vi "Lift State Machine.vi"() -> ()   [LabVIEW 2014]
uses:
  Global Variables.vi
panel:
  in  "Lift Speed 2":dbl=0.25 format="%#_13g"
  in  "Distance Down":dbl=6.0 format="%#_13g"
  in  "Distance Back Up":dbl=6.0 format="%#_13g"
  in  "Lift Speed":dbl=3.0
  in  "Offset":u32=3
  in  "Offset Step":bool
  out "State":i32=3
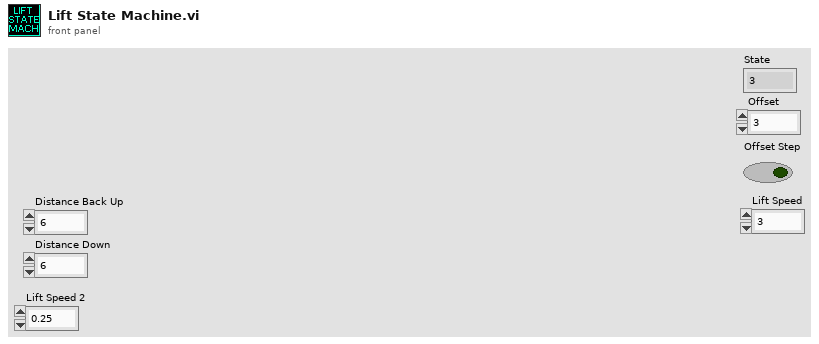
[diagram p1: front panel]
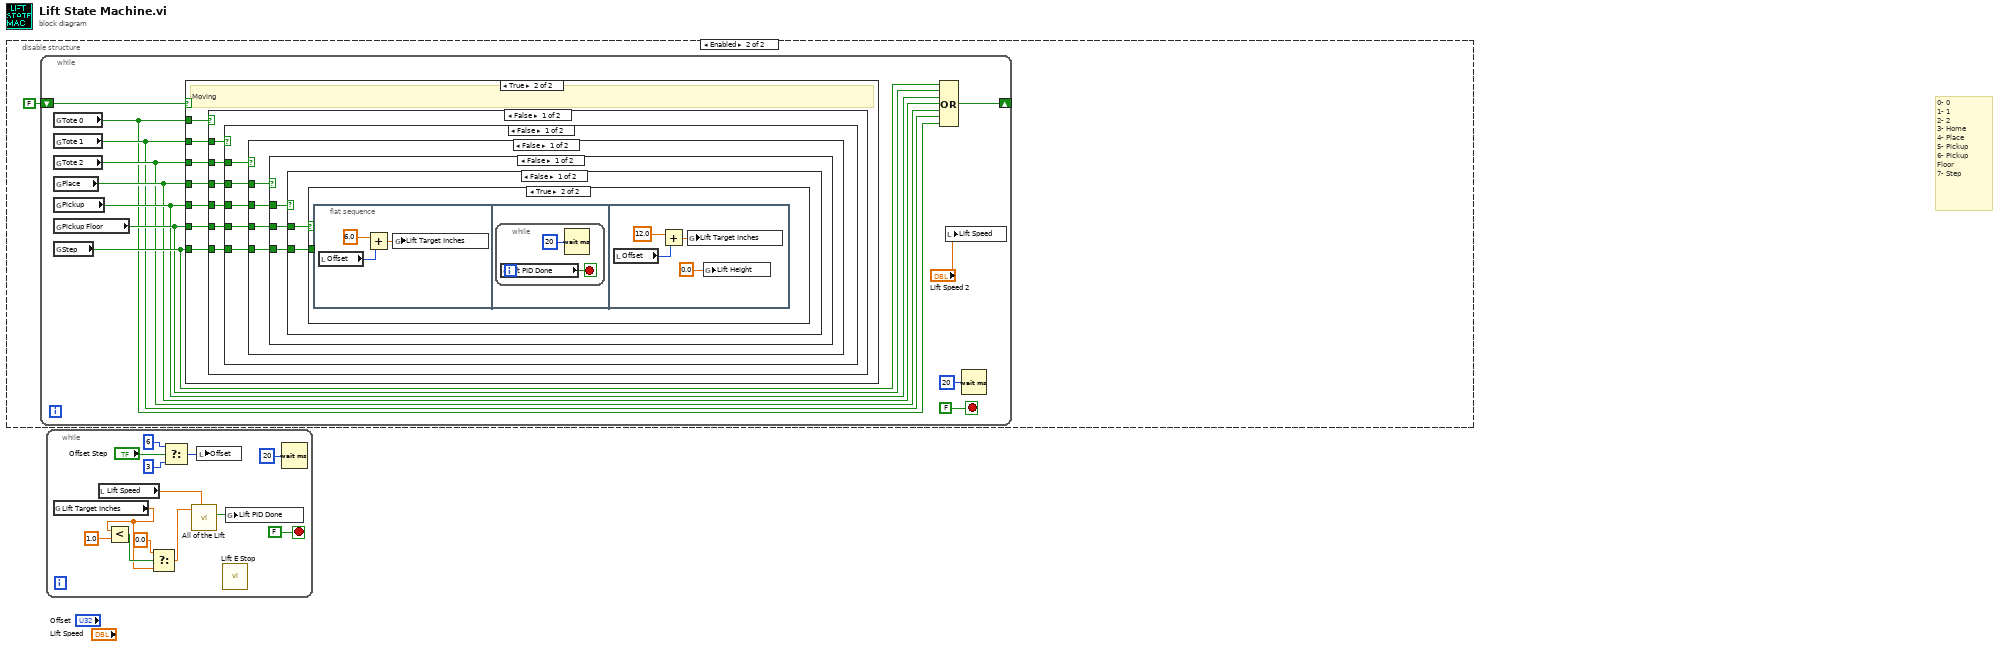
[diagram p0: block diagram]
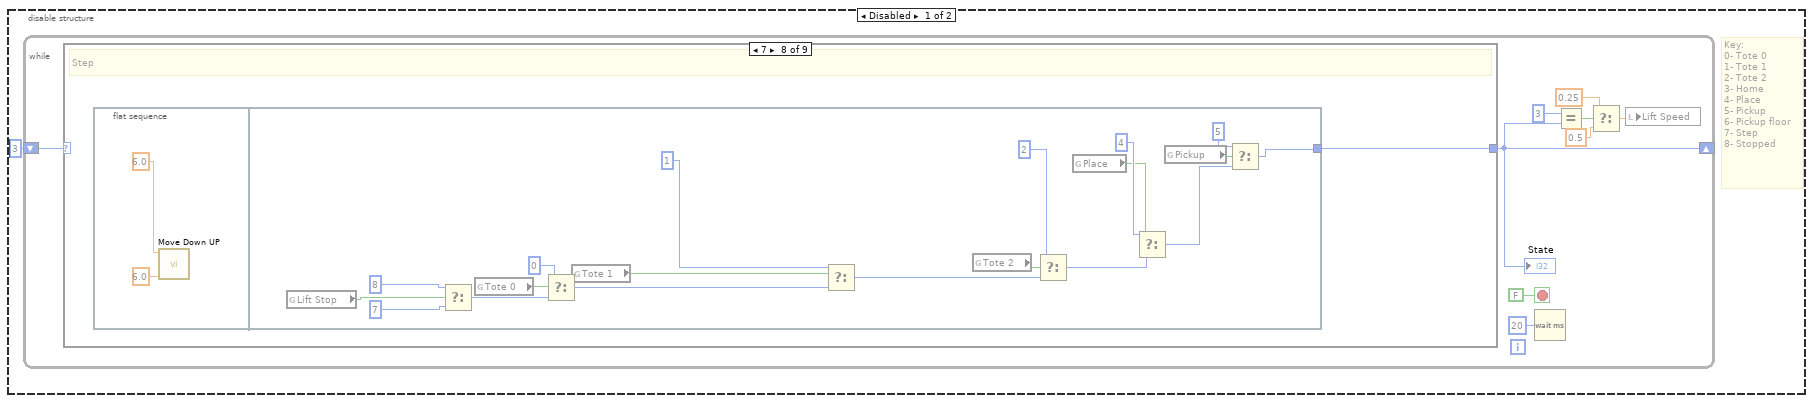
[diagram p2: hidden frame]
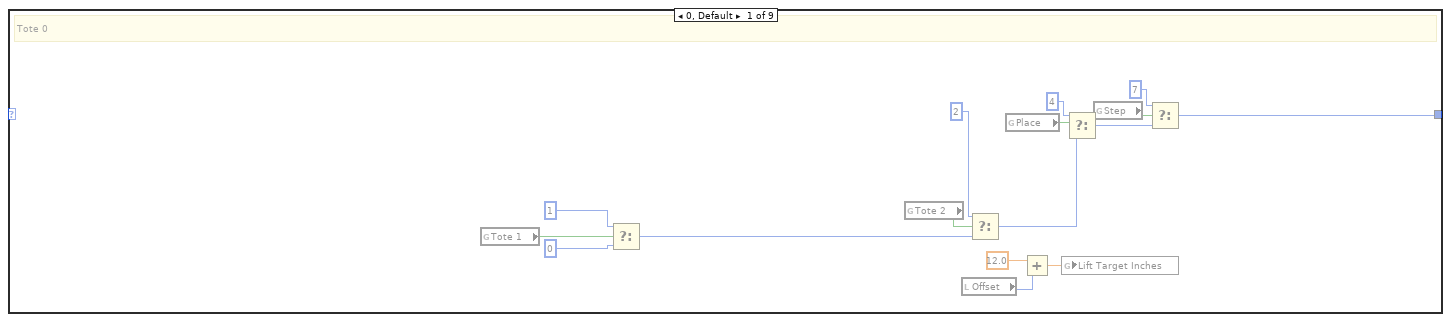
[diagram p3: hidden frame]
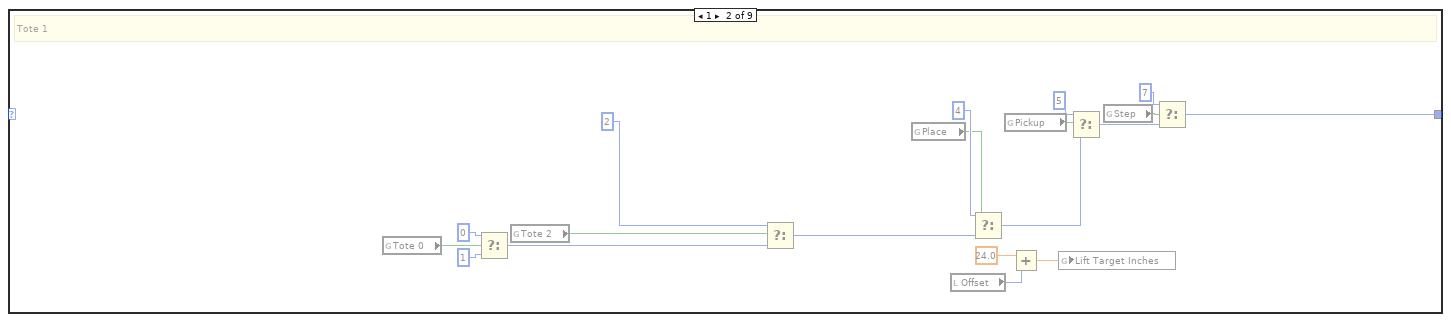
[diagram p4: hidden frame]
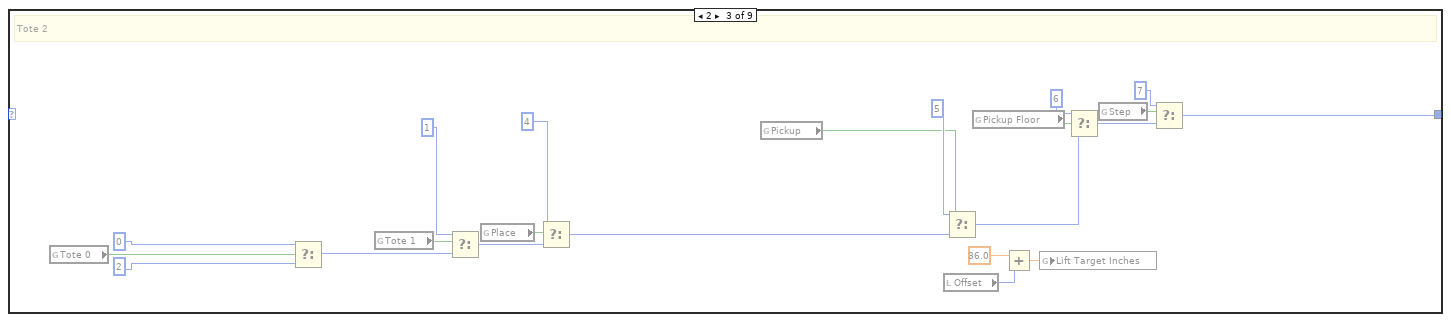
[diagram p5: hidden frame]
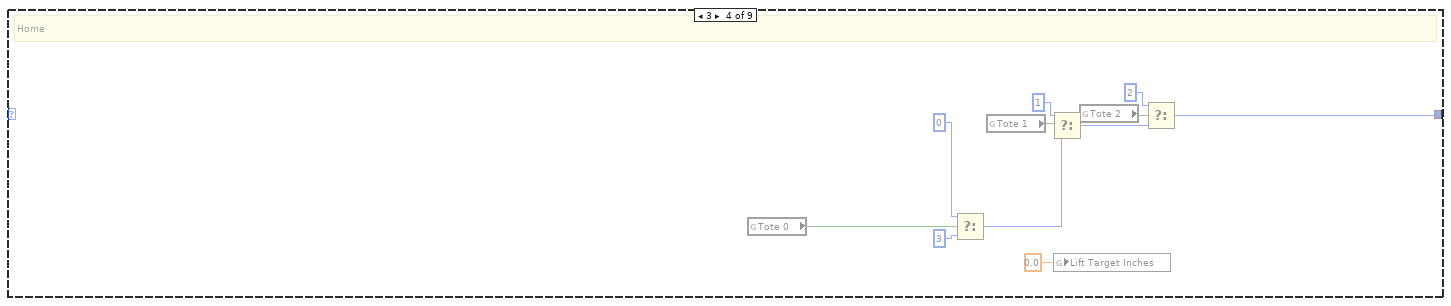
[diagram p6: hidden frame]
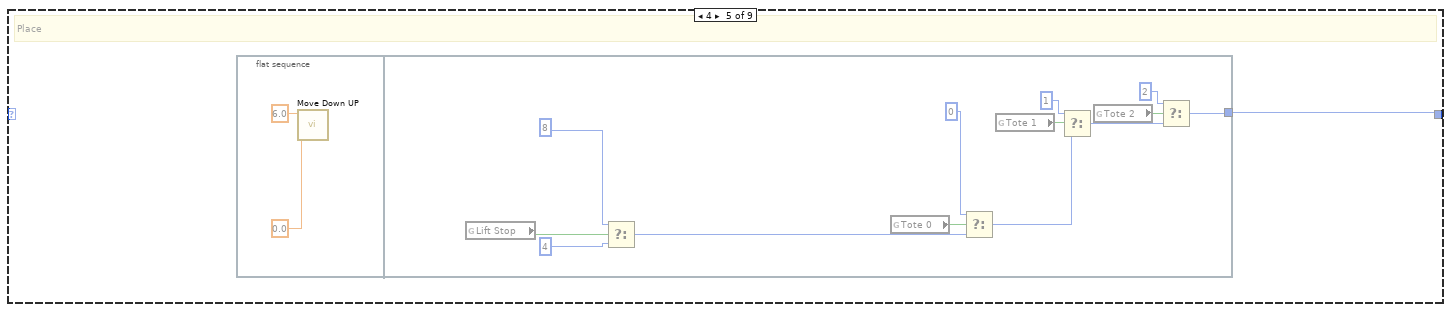
[diagram p7: hidden frame]
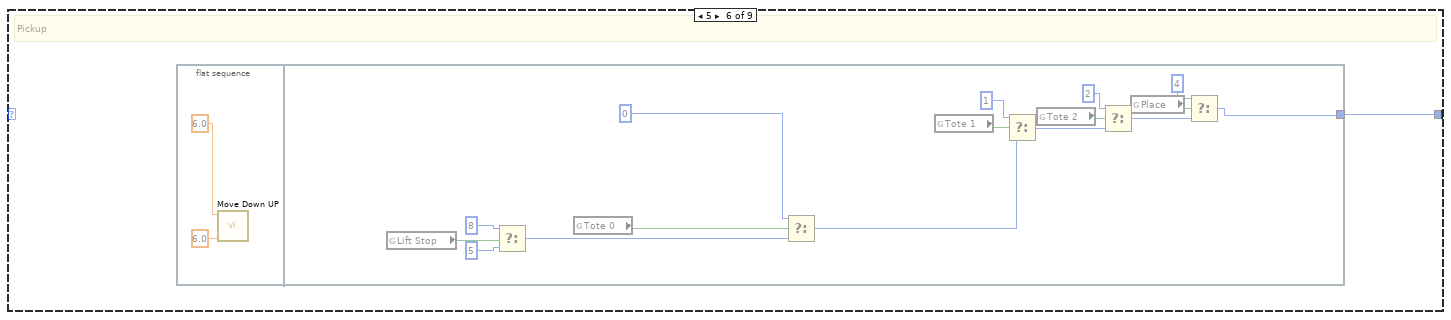
[diagram p8: hidden frame]
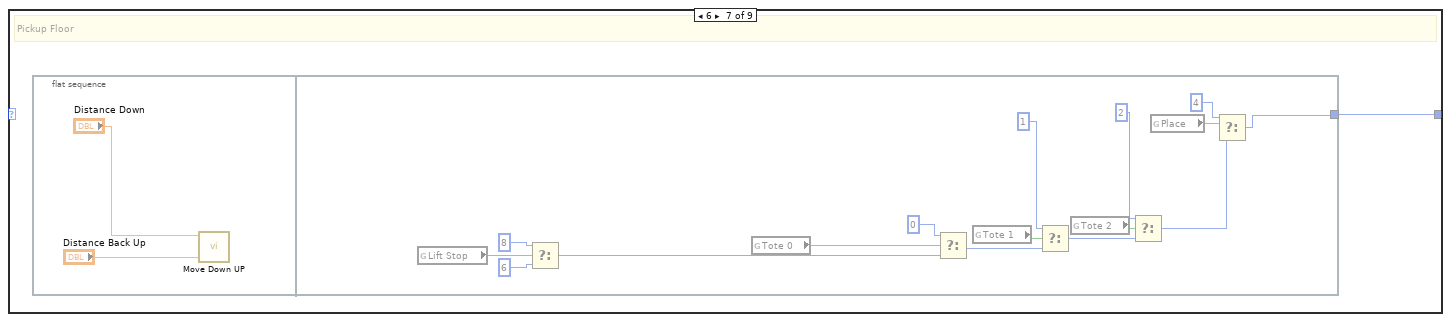
[diagram p9: hidden frame]
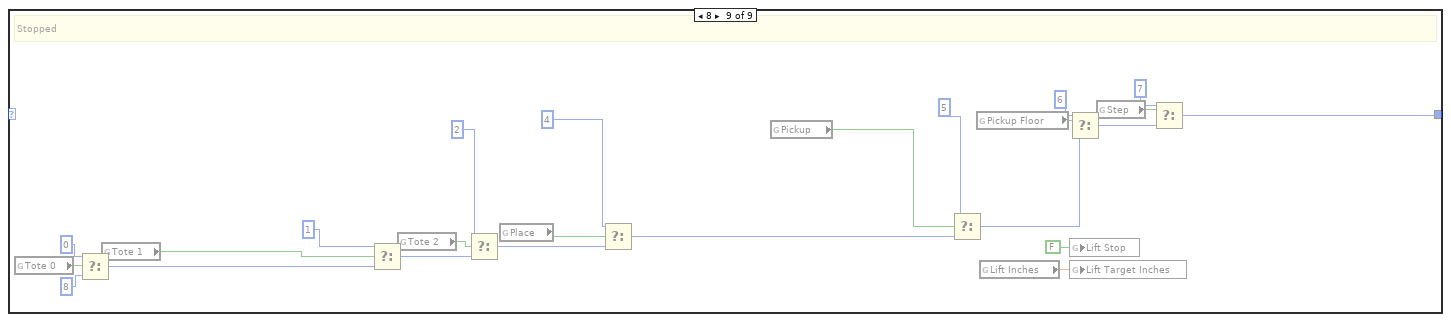
[diagram p10: hidden frame]
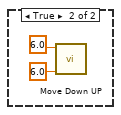
[diagram p13: hidden frame]
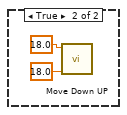
[diagram p14: hidden frame]
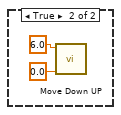
[diagram p15: hidden frame]
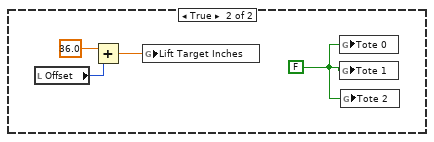
[diagram p16: hidden frame]
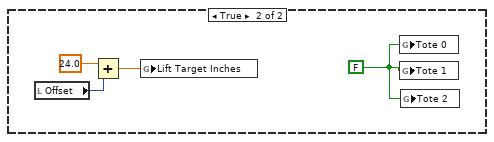
[diagram p17: hidden frame]
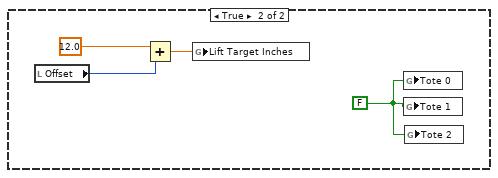
[diagram p18: hidden frame]
diagram:
  # "0- 0\n1- 1\n2- 2\n3- Home\n4- Place\n5- Pickup\n6- Pickup Floor\n7- Step"
  n1 = disable-structure shown="Enabled" {
    frame Disabled {
      # "Key:\n0- Tote 0\n1- Tote 1\n2- Tote 2\n3- Home\n4- Place\n5- Pickup\n6- Pickup floor\n7- Step\n8- Stopped"
      n2 = while {
        shift-right: [w6] -> _
        shift-left: 3 ("f") -> [w10]
        stop <- FALSE stop-if-true
        n3 = case shown="7" w10 {
          tunnel: [w19 w40 w63 w72 w79 w95 w114 w133 w156] -> w6
          frame 0, Default {
            # "Tote 0"
            n4 = global read "Global Variables.vi" "Tote 1"() -> (w15:bool)
            n5 = Select(t=1, s=w15, f=0) -> (s? t:f=w23:i32)
            n6 = global read "Global Variables.vi" "Tote 2"() -> (w14:bool)
            n7 = local read "Offset"() -> (w16:u32)
            n8 = Select(t=2, s=w14, f=w23) -> (s? t:f=w20:i32)
            n9 = global read "Global Variables.vi" "Place"() -> (w13:bool)
            n10 = Add(x=12.0, y=w16) -> (x+y=w11:dbl)
            n11 = global write "Global Variables.vi" "Lift Target Inches"(w11) -> ()
            n12 = Select(t=4, s=w13, f=w20) -> (s? t:f=w18:i32)
            n13 = global read "Global Variables.vi" "Step"() -> (w12:bool)
            n14 = Select(t=7, s=w12, f=w18) -> (s? t:f=w19:i32)
          }
          frame 1 {
            # "Tote 1"
            n15 = global read "Global Variables.vi" "Tote 0"() -> (w32:bool)
            n16 = Select(t=0, s=w32, f=1) -> (s? t:f=w37:i32)
            n17 = global read "Global Variables.vi" "Tote 2"() -> (w31:bool)
            n18 = Select(t=2, s=w31, f=w37) -> (s? t:f=w36:i32)
            n19 = global read "Global Variables.vi" "Place"() -> (w30:bool)
            n20 = local read "Offset"() -> (w33:u32)
            n21 = Select(t=4, s=w30, f=w36) -> (s? t:f=w39:i32)
            n22 = global read "Global Variables.vi" "Pickup"() -> (w29:bool)
            n23 = Add(x=24.0, y=w33) -> (x+y=w27:dbl)
            n24 = global write "Global Variables.vi" "Lift Target Inches"(w27) -> ()
            n25 = Select(t=5, s=w29, f=w39) -> (s? t:f=w35:i32)
            n26 = global read "Global Variables.vi" "Step"() -> (w28:bool)
            n27 = Select(t=7, s=w28, f=w35) -> (s? t:f=w40:i32)
          }
          frame 2 {
            # "Tote 2"
            n28 = global read "Global Variables.vi" "Tote 0"() -> (w53:bool)
            n29 = Select(t=0, s=w53, f=2) -> (s? t:f=w61:i32)
            n30 = global read "Global Variables.vi" "Tote 1"() -> (w52:bool)
            n31 = Select(t=1, s=w52, f=w61) -> (s? t:f=w59:i32)
            n32 = global read "Global Variables.vi" "Place"() -> (w48:bool)
            n33 = Select(t=4, s=w48, f=w59) -> (s? t:f=w57:i32)
            n34 = global read "Global Variables.vi" "Pickup"() -> (w47:bool)
            n35 = local read "Offset"() -> (w54:u32)
            n36 = Select(t=5, s=w47, f=w57) -> (s? t:f=w56:i32)
            n37 = global read "Global Variables.vi" "Pickup Floor"() -> (w51:bool)
            n38 = Add(x=36.0, y=w54) -> (x+y=w49:dbl)
            n39 = global write "Global Variables.vi" "Lift Target Inches"(w49) -> ()
            n40 = Select(t=6, s=w51, f=w56) -> (s? t:f=w66:i32)
            n41 = global read "Global Variables.vi" "Step"() -> (w50:bool)
            n42 = Select(t=7, s=w50, f=w66) -> (s? t:f=w63:i32)
          }
          frame 3 {
            # "Home"
            n43 = global read "Global Variables.vi" "Tote 0"() -> (w71:bool)
            n44 = Select(t=0, s=w71, f=3) -> (s? t:f=w74:i32)
            n45 = global read "Global Variables.vi" "Tote 1"() -> (w70:bool)
            n46 = Select(t=1, s=w70, f=w74) -> (s? t:f=w77:i32)
            n47 = global write "Global Variables.vi" "Lift Target Inches"(0.0 ("x")) -> ()
            n48 = global read "Global Variables.vi" "Tote 2"() -> (w69:bool)
            n49 = Select(t=2, s=w69, f=w77) -> (s? t:f=w72:i32)
          }
          frame 4 {
            # "Place"
            n50 = flat-sequence {
              tunnel: [w82] -> w79
              frame #0 {
                n51 = call "Move Down UP.vi"("Distance Up"=0.0, "Distance Down"=6.0) -> ()  [unwired: 10 in]
              }
              frame #1 {
                n52 = global read "Global Variables.vi" "Lift Stop"() -> (w86:bool)
                n53 = Select(t=8, s=w86, f=4) -> (s? t:f=w83:i32)
                n54 = global read "Global Variables.vi" "Tote 0"() -> (w89:bool)
                n55 = Select(t=0, s=w89, f=w83) -> (s? t:f=w91:i32)
                n56 = global read "Global Variables.vi" "Tote 1"() -> (w88:bool)
                n57 = Select(t=1, s=w88, f=w91) -> (s? t:f=w93:i32)
                n58 = global read "Global Variables.vi" "Tote 2"() -> (w87:bool)
                n59 = Select(t=2, s=w87, f=w93) -> (s? t:f=w82:i32)
              }
            }
          }
          frame 5 {
            # "Pickup"
            n60 = flat-sequence {
              tunnel: [w98] -> w95
              frame #0 {
                n61 = call "Move Down UP.vi"("Distance Up"=6.0, "Distance Down"=6.0) -> ()  [unwired: 10 in]
              }
              frame #1 {
                n62 = global read "Global Variables.vi" "Lift Stop"() -> (w102:bool)
                n63 = Select(t=8, s=w102, f=5) -> (s? t:f=w99:i32)
                n64 = global read "Global Variables.vi" "Tote 0"() -> (w106:bool)
                n65 = Select(t=0, s=w106, f=w99) -> (s? t:f=w107:i32)
                n66 = global read "Global Variables.vi" "Tote 1"() -> (w105:bool)
                n67 = Select(t=1, s=w105, f=w107) -> (s? t:f=w110:i32)
                n68 = global read "Global Variables.vi" "Tote 2"() -> (w104:bool)
                n69 = Select(t=2, s=w104, f=w110) -> (s? t:f=w109:i32)
                n70 = global read "Global Variables.vi" "Place"() -> (w103:bool)
                n71 = Select(t=4, s=w103, f=w109) -> (s? t:f=w98:i32)
              }
            }
          }
          frame 6 {
            # "Pickup Floor"
            n72 = flat-sequence {
              tunnel: [w118] -> w114
              frame #0 {
                n73 = call "Move Down UP.vi"("Distance Up"="Distance Back Up", "Distance Down"="Distance Down") -> ()  [unwired: 10 in]
              }
              frame #1 {
                n74 = global read "Global Variables.vi" "Lift Stop"() -> (w119:bool)
                n75 = Select(t=8, s=w119, f=6) -> (s? t:f=w120:i32)
                n76 = global read "Global Variables.vi" "Tote 0"() -> (w126:bool)
                n77 = Select(t=0, s=w126, f=w120) -> (s? t:f=w127:i32)
                n78 = global read "Global Variables.vi" "Tote 1"() -> (w125:bool)
                n79 = Select(t=1, s=w125, f=w127) -> (s? t:f=w130:i32)
                n80 = global read "Global Variables.vi" "Tote 2"() -> (w124:bool)
                n81 = Select(t=2, s=w124, f=w130) -> (s? t:f=w129:i32)
                n82 = global read "Global Variables.vi" "Place"() -> (w123:bool)
                n83 = Select(t=4, s=w123, f=w129) -> (s? t:f=w118:i32)
              }
            }
          }
          frame 7 {
            # "Step"
            n84 = flat-sequence {
              tunnel: [w136] -> w133
              frame #0 {
                n85 = call "Move Down UP.vi"("Distance Up"=6.0, "Distance Down"=6.0) -> ()  [unwired: 10 in]
              }
              frame #1 {
                n86 = global read "Global Variables.vi" "Lift Stop"() -> (w137:bool)
                n87 = Select(t=8, s=w137, f=7) -> (s? t:f=w139:i32)
                n88 = global read "Global Variables.vi" "Tote 0"() -> (w145:bool)
                n89 = Select(t=0, s=w145, f=w139) -> (s? t:f=w146:i32)
                n90 = global read "Global Variables.vi" "Tote 1"() -> (w144:bool)
                n91 = Select(t=1, s=w144, f=w146) -> (s? t:f=w150:i32)
                n92 = global read "Global Variables.vi" "Tote 2"() -> (w143:bool)
                n93 = Select(t=2, s=w143, f=w150) -> (s? t:f=w151:i32)
                n94 = global read "Global Variables.vi" "Place"() -> (w142:bool)
                n95 = Select(t=4, s=w142, f=w151) -> (s? t:f=w148:i32)
                n96 = global read "Global Variables.vi" "Pickup"() -> (w141:bool)
                n97 = Select(t=5, s=w141, f=w148) -> (s? t:f=w136:i32)
              }
            }
          }
          frame 8 {
            # "Stopped"
            n98 = global read "Global Variables.vi" "Tote 0"() -> (w158:bool)
            n99 = Select(t=0, s=w158, f=8) -> (s? t:f=w160:i32)
            n100 = global read "Global Variables.vi" "Tote 1"() -> (w163:bool)
            n101 = Select(t=1, s=w163, f=w160) -> (s? t:f=w161:i32)
            n102 = global read "Global Variables.vi" "Tote 2"() -> (w168:bool)
            n103 = Select(t=2, s=w168, f=w161) -> (s? t:f=w169:i32)
            n104 = global read "Global Variables.vi" "Place"() -> (w167:bool)
            n105 = Select(t=4, s=w167, f=w169) -> (s? t:f=w173:i32)
            n106 = global read "Global Variables.vi" "Pickup"() -> (w166:bool)
            n107 = Select(t=5, s=w166, f=w173) -> (s? t:f=w174:i32)
            n108 = global read "Global Variables.vi" "Pickup Floor"() -> (w165:bool)
            n109 = global read "Global Variables.vi" "Lift Inches"() -> (w178:dbl)
            n110 = Select(t=6, s=w165, f=w174) -> (s? t:f=w171:i32)
            n111 = global write "Global Variables.vi" "Lift Stop"(FALSE ("Lift Stop")) -> ()
            n112 = global write "Global Variables.vi" "Lift Target Inches"(w178) -> ()
            n113 = global read "Global Variables.vi" "Step"() -> (w164:bool)
            n114 = Select(t=7, s=w164, f=w171) -> (s? t:f=w156:i32)
          }
        }
        "State" <- w6
        n115 = Wait (ms)(milliseconds to wait=u32 20) -> ()  [unwired: 1 out]
        n116 = Equal?(x=3, y=w6) -> (x = y?=w5:bool)
        n117 = Select(t=0.25, s=w5, f=0.5) -> (s? t:f=w7:dbl)
        n118 = local write "Lift Speed"(w7) -> ()
      }
    }
    frame Enabled {
      n119 = while {
        shift-right: [w182] -> _
        shift-left: FALSE -> [w190]
        stop <- FALSE stop-if-true
        n120 = global read "Global Variables.vi" "Tote 0"() -> (w183:bool)
        n121 = global read "Global Variables.vi" "Tote 1"() -> (w184:bool)
        n122 = global read "Global Variables.vi" "Tote 2"() -> (w185:bool)
        n123 = global read "Global Variables.vi" "Place"() -> (w186:bool)
        n124 = global read "Global Variables.vi" "Pickup"() -> (w187:bool)
        n125 = global read "Global Variables.vi" "Pickup Floor"() -> (w188:bool)
        n126 = global read "Global Variables.vi" "Step"() -> (w189:bool)
        n127 = case shown="True" w190 {
          tunnel: w183 -> [_ w198]
          tunnel: w184 -> [_ w197]
          tunnel: w185 -> [_ w196]
          tunnel: w186 -> [_ w195]
          tunnel: w187 -> [_ w194]
          tunnel: w188 -> [_ w193]
          tunnel: w189 -> [_ w192]
          frame False {
            # "Idling"
          }
          frame True {
            # "Moving"
            n128 = case shown="False" w198 {
              tunnel: w197 -> [w204 _]
              tunnel: w196 -> [w203 _]
              tunnel: w195 -> [w202 _]
              tunnel: w194 -> [w201 _]
              tunnel: w193 -> [w200 _]
              tunnel: w192 -> [w199 _]
              frame False {
                n129 = case shown="False" w204 {
                  tunnel: w203 -> [w209 _]
                  tunnel: w202 -> [w208 _]
                  tunnel: w201 -> [w207 _]
                  tunnel: w200 -> [w206 _]
                  tunnel: w199 -> [w205 _]
                  frame False {
                    n130 = case shown="False" w209 {
                      tunnel: w208 -> [w213 _]
                      tunnel: w207 -> [w212 _]
                      tunnel: w206 -> [w211 _]
                      tunnel: w205 -> [w210 _]
                      frame False {
                        n131 = case shown="False" w213 {
                          tunnel: w212 -> [w216 _]
                          tunnel: w211 -> [w215 _]
                          tunnel: w210 -> [w214 _]
                          frame False {
                            n132 = case shown="False" w216 {
                              tunnel: w215 -> [w218 _]
                              tunnel: w214 -> [w217 _]
                              frame False {
                                n133 = case shown="True" w218 {
                                tunnel: w217 -> [w219 _]
                                frame False {
                                n134 = case shown="False" w219 {
                                frame False {
                                }
                                frame True {
                                n135 = call "Move Down UP.vi"("Distance Up"=6.0, "Distance Down"=6.0) -> ()  [unwired: 10 in]
                                }
                                }
                                }
                                frame True {
                                n136 = flat-sequence {
                                frame #0 {
                                n137 = local read "Offset"() -> (w223:u32)
                                n138 = Add(x=6.0, y=w223) -> (x+y=w224:dbl)
                                n139 = global write "Global Variables.vi" "Lift Target Inches"(w224) -> ()
                                }
                                frame #1 {
                                n140 = while {
                                stop <- w226 stop-if-true
                                n141 = global read "Global Variables.vi" "Lift PID Done"() -> (w226:bool)
                                n142 = Wait (ms)(milliseconds to wait=u32 20) -> ()  [unwired: 1 out]
                                }
                                }
                                frame #2 {
                                n143 = local read "Offset"() -> (w229:u32)
                                n144 = Add(x=12.0, y=w229) -> (x+y=w230:dbl)
                                n145 = global write "Global Variables.vi" "Lift Target Inches"(w230) -> ()
                                n146 = global write "Global Variables.vi" "Lift Height"(0.0 ("Lift Target Inches")) -> ()
                                }
                                }
                                }
                                }
                              }
                              frame True {
                                n147 = call "Move Down UP.vi"("Distance Up"=18.0, "Distance Down"=18.0) -> ()  [unwired: 10 in]
                              }
                            }
                          }
                          frame True {
                            n148 = call "Move Down UP.vi"("Distance Up"=0.0, "Distance Down"=6.0) -> ()  [unwired: 10 in]
                          }
                        }
                      }
                      frame True {
                        w235 = FALSE
                        n149 = local read "Offset"() -> (w237:u32)
                        n150 = Add(x=36.0, y=w237) -> (x+y=w238:dbl)
                        n151 = global write "Global Variables.vi" "Lift Target Inches"(w238) -> ()
                        n152 = global write "Global Variables.vi" "Tote 0"(w235) -> ()
                        n153 = global write "Global Variables.vi" "Tote 1"(w235) -> ()
                        n154 = global write "Global Variables.vi" "Tote 2"(w235) -> ()
                      }
                    }
                  }
                  frame True {
                    w239 = FALSE
                    n155 = local read "Offset"() -> (w241:u32)
                    n156 = Add(x=24.0, y=w241) -> (x+y=w242:dbl)
                    n157 = global write "Global Variables.vi" "Lift Target Inches"(w242) -> ()
                    n158 = global write "Global Variables.vi" "Tote 0"(w239) -> ()
                    n159 = global write "Global Variables.vi" "Tote 1"(w239) -> ()
                    n160 = global write "Global Variables.vi" "Tote 2"(w239) -> ()
                  }
                }
              }
              frame True {
                w243 = FALSE
                n161 = local read "Offset"() -> (w245:u32)
                n162 = Add(x=12.0, y=w245) -> (x+y=w246:dbl)
                n163 = global write "Global Variables.vi" "Lift Target Inches"(w246) -> ()
                n164 = global write "Global Variables.vi" "Tote 0"(w243) -> ()
                n165 = global write "Global Variables.vi" "Tote 1"(w243) -> ()
                n166 = global write "Global Variables.vi" "Tote 2"(w243) -> ()
              }
            }
          }
        }
        n167 = Compound Arithmetic op=OR(w189, w188, w187, w186, w185, w184, w183) -> (w182:bool)
        n168 = local write "Lift Speed"("Lift Speed 2") -> ()
        n169 = Wait (ms)(milliseconds to wait=u32 20) -> ()  [unwired: 1 out]
      }
    }
  }
  n170 = while {
    stop <- FALSE stop-if-true
    n171 = global read "Global Variables.vi" "Lift Target Inches"() -> (w248:dbl)
    n172 = local read "Lift Speed"() -> (w252:dbl)
    n173 = Less?(x=w248, y=1.0) -> (x < y?=w251:bool)
    n174 = Select(t=0.0, s=w251, f=w248) -> (s? t:f=w250:dbl)
    n175 = Select(t=6, s="Offset Step", f=3) -> (s? t:f=w254:i32)
    n176 = call "All of the Lift.vi"("Speed"=w252, "Inches to move"=w250) -> ("Done"=w259:bool)  [unwired: 9 in]
    n177 = local write "Offset"(w254) -> ()
    n178 = call "Lift E Stop.vi"() -> ()  [unwired: 12 in]
    n179 = global write "Global Variables.vi" "Lift PID Done"(w259) -> ()
    n180 = Wait (ms)(milliseconds to wait=u32 20) -> ()  [unwired: 1 out]
  }
